vi "ReadVSChCyclicOutgoing.vi"(7 "CyclicFRActive?":bool, 8 "error in (no error)":errorcluster, 9 "Input Values in":dbl[](array[numeric]), 10 "Input Refs":T1[](array[typedef]) format="%.0x", 11 "Refnum in":refnum<k21>) -> (0 "error out":errorcluster, 1 "Input Values out":dbl[](array[numeric]), 3 "Refnum out":refnum<k21>)   [LabVIEW 2020, in "FlexRay Custom Device Engine.lvlib"]
uses:
  FlexRay Custom Device Engine.lvlib
  <vilib>/NI VeriStand/Custom Device API/Data Reference.ctl
  <vilib>/NI VeriStand/Custom Device API/Global Data Refs.vi
  <vilib>/xnet/xnet.llb/XNET Write (Signal Single-point).vi
  <vilib>/NI VeriStand/Custom Device API/Custom Device API.lvlib
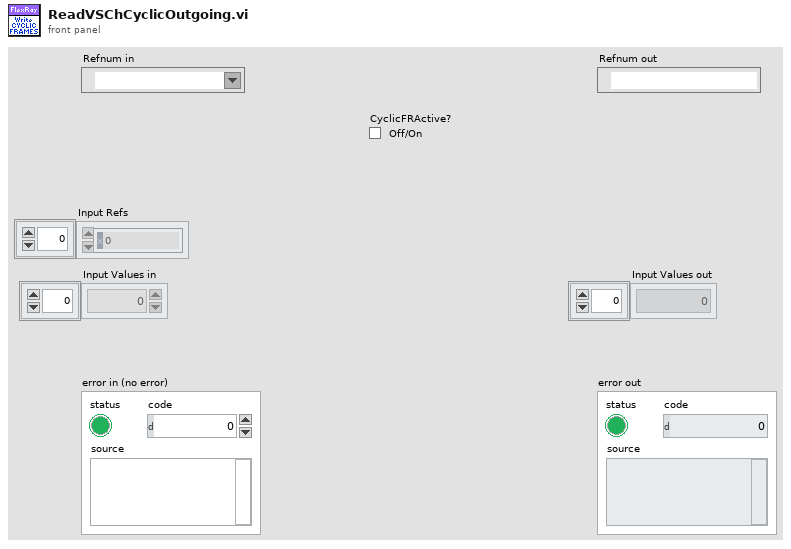
[diagram p1: front panel]
types:
  T1 = typedef "Custom Device API.lvlib/Data Reference.ctl" = i32
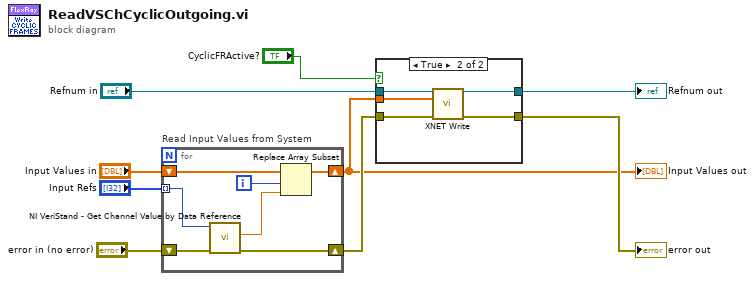
[diagram p0: block diagram]
diagram:
  n1 = for "Read Input Values from System" {
    shift-right: [w10] -> w3
    shift-left: "error in (no error)" -> [w16]
    tunnel: "Input Refs" -> [w15] mode=indexing
    shift-right: [w13] -> w2
    shift-left: "Input Values in" -> [w14]
    i -> [w12]
    n2 = call <vilib>:"NI VeriStand - Get Channel Value by Data Reference.vi"("error in (no error)"=w16, "Data Reference in"=w15) -> ("error out"=w10:errorcluster, "Value"=w11:dbl)  [unwired: 8 out]
    n3 = Replace Array Subset(array=w14, new element=w11, index=w12) -> (w13:dbl[])
  }
  "Input Values out" <- w2
  n4 = case shown="True" "CyclicFRActive?" {
    tunnel: w2 -> [_ w23]
    tunnel: w3 -> [w17 w22]
    tunnel: [w17 w21] -> w4
    tunnel: "Refnum in" -> [w18 w20]
    tunnel: [w18 w19] -> w7
    frame False {
    }
    frame True {
      n5 = call-poly <vilib>:"XNET Write.vi"("session in"=w20, "data"=w23, "error in (no error)"=w22) -> ("session out"=w19:refnum<k21>, "error out"=w21:errorcluster)  [unwired: 11 in]
    }
  }
  "Refnum out" <- w7
  "error out" <- w4
